vi "TIFKATS Command.vi"(7 "Description":string, 8 "Command Info In":T2, 10 "Setpoint":dbl, 11 "Operation":T1) -> (0 "Command Info Out":T2)   [LabVIEW 2023]
doc: "This template is useful for immediate subsystem actions that do not need deadband filtering\n\nBe sure to right-click and select New from Template and save with a new command name."
uses:
  <vilib>/Rock Robotics/WPI/Framework/Command Status Info.ctl
  <vilib>/Rock Robotics/WPI/Framework/Completion Status.ctl
  <vilib>/Rock Robotics/WPI/Framework/Completion Notifier.ctl
  Implementation/TIFKATS Operations.ctl
  Implementation/TIFKATS Setpoints2c.ctl
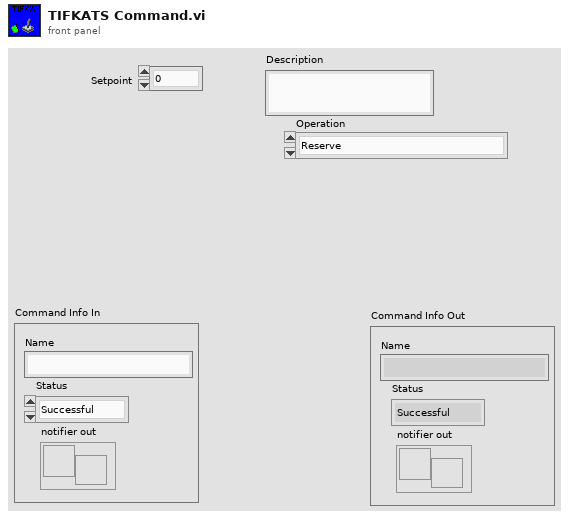
[diagram p1: front panel]
types:
  T1 = typedef "TIFKATS Operations.ctl" = enum16{"Reserve", "Read Current", "Immediate", "Load", "Amp", "Shoot", "Intake", "Spit", "Stop All"}
  T2 = typedef "Command Status Info.ctl" = cluster{"Name":string, "Status":T3, "notifier out":T4}
  T3 = typedef "Completion Status.ctl" = enum16{"Successful", "Aborted", "Incomplete"}
  T4 = typedef "Completion Notifier.ctl" = refnum<notifier>
  T5 = typedef "TIFKATS Setpoints2c.ctl" = cluster{"Operation":T1, "Angle":dbl}
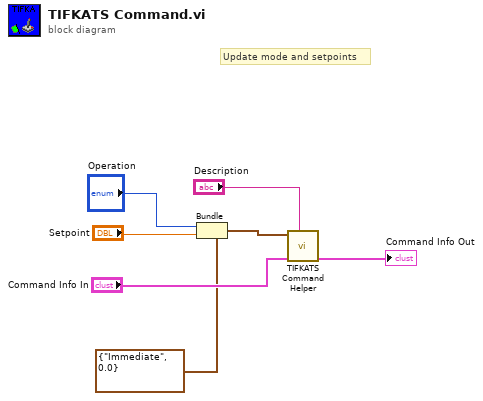
[diagram p0: block diagram]
diagram:
  # "Update mode and setpoints"
  n1 = Bundle(cluster=T5 {"Operation"=enum."Immediate", "Angle"=0.0} ("SubSystem Data"), "Operation"="Operation", "Angle"="Setpoint") -> (w2:T5)
  n2 = call "TIFKATS Command Helper.vi"("Description"="Description", "Command Info In"="Command Info In", "SubSystem Data"=w2) -> ("Command Info Out"=→"Command Info Out":T2)  [unwired: 6 in, 2 out]
